vi "AlAs-GaAs superlattice-111230a.vi"() -> ()   [LabVIEW 2011]
uses:
  wait_globals.vi
panel:
  out "Total Wait Time (m:s)":string
  out "step number  2":i32
  in  "Number of \nGrowth Steps 6":i32=20
  out "Wait Time Remaining(m:s)":string
  out "Waiting":bool
  in  "Ga Flow 1":dbl=5.49
  in  "Aluminum Flow":dbl=10.0
  in  "Number of \nGrowth Steps":i32=20
  out "step number":i32
  in  "As_Gas Flow":dbl=3.4
  in  "Manifold H2 Flow":dbl=730.0
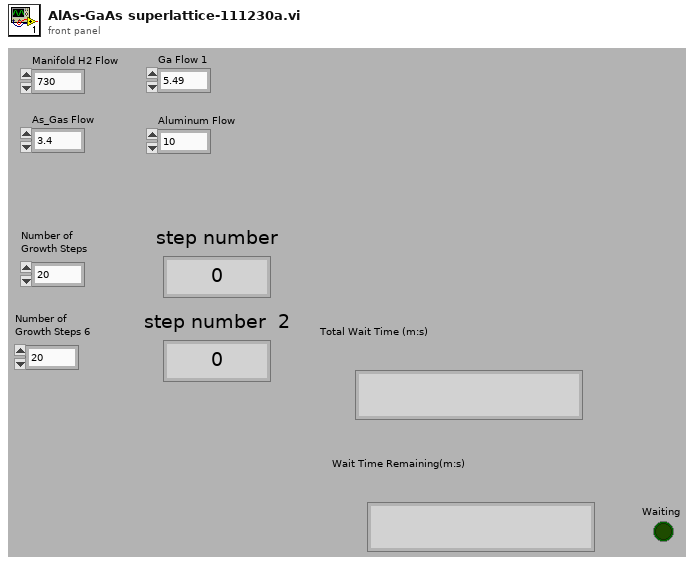
[diagram p1: front panel]
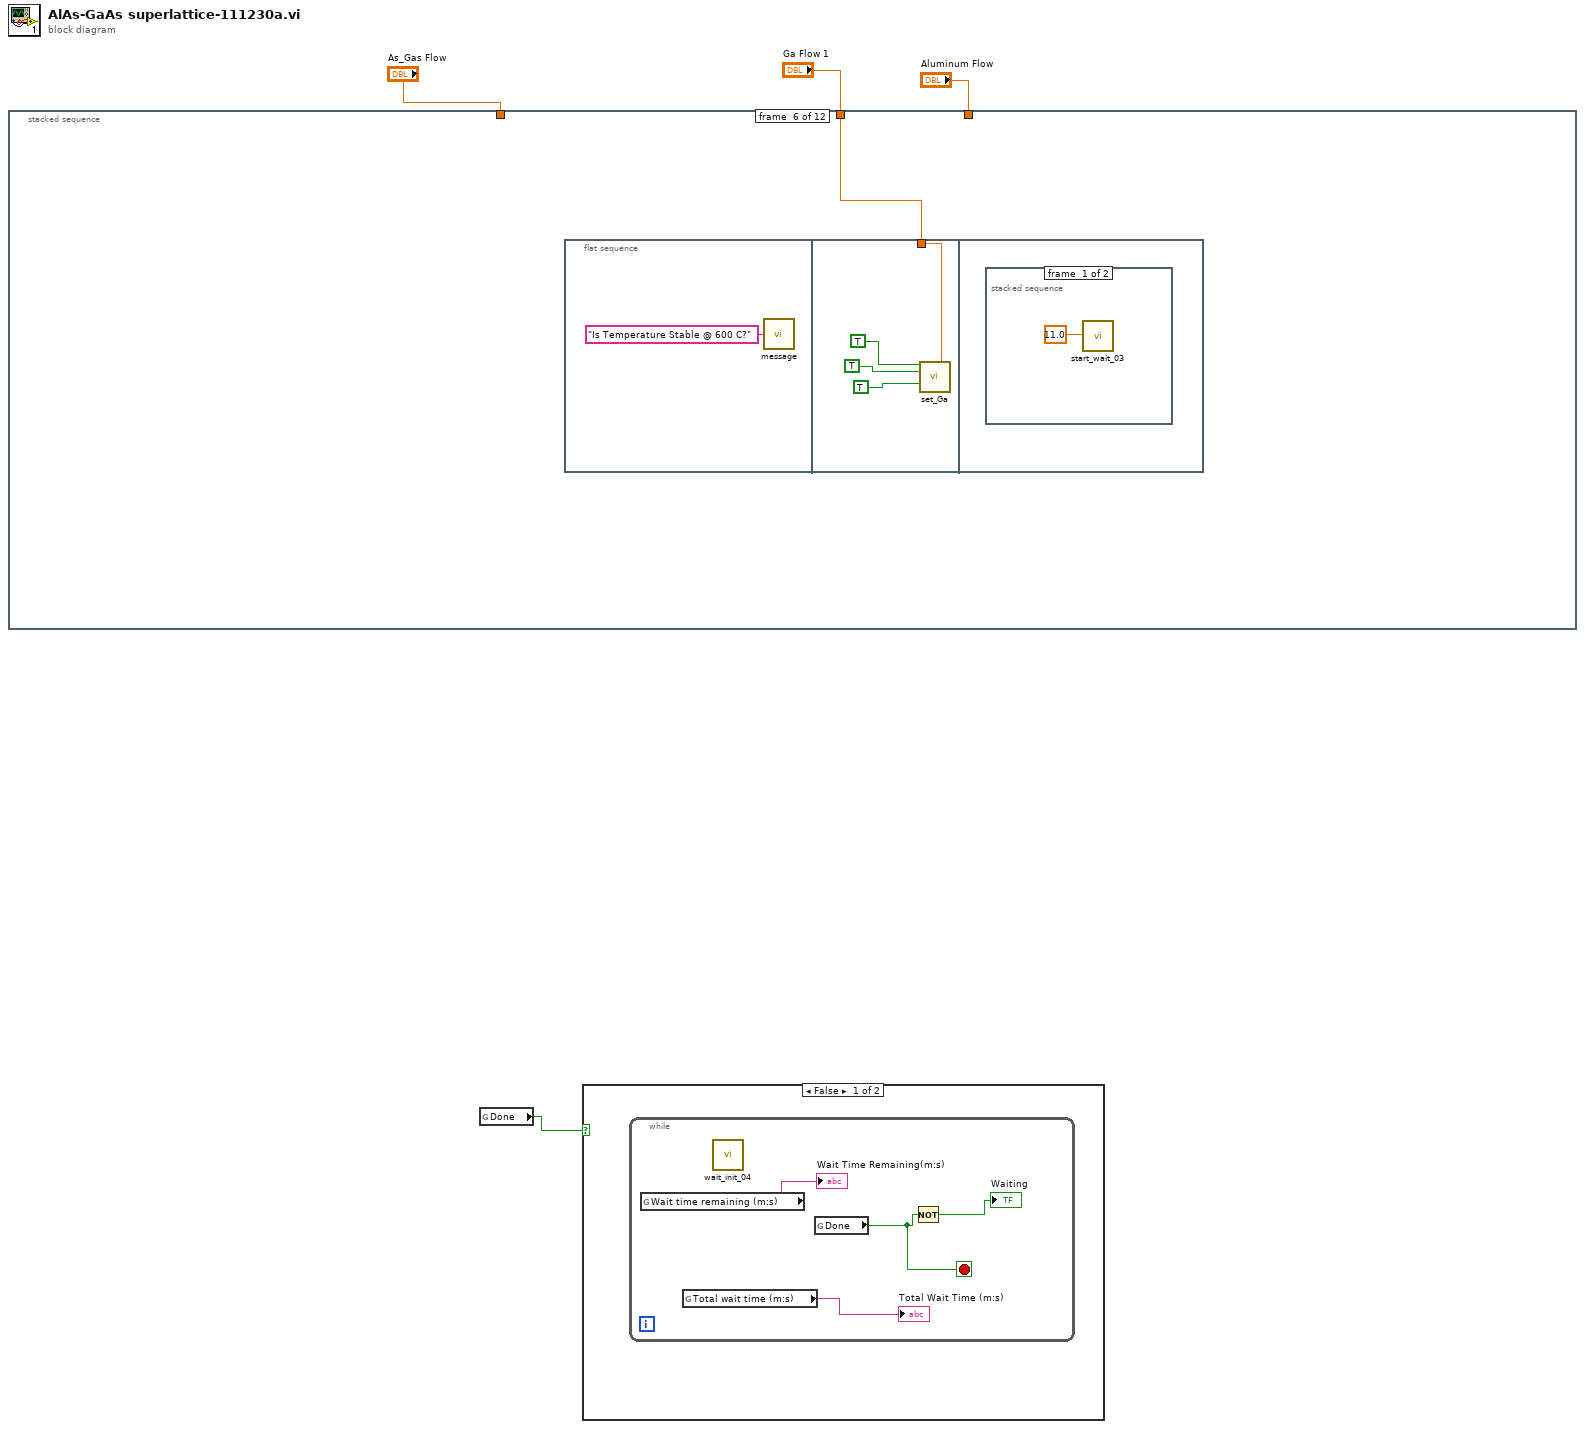
[diagram p0: block diagram]
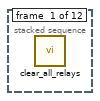
[diagram p3: hidden frame]
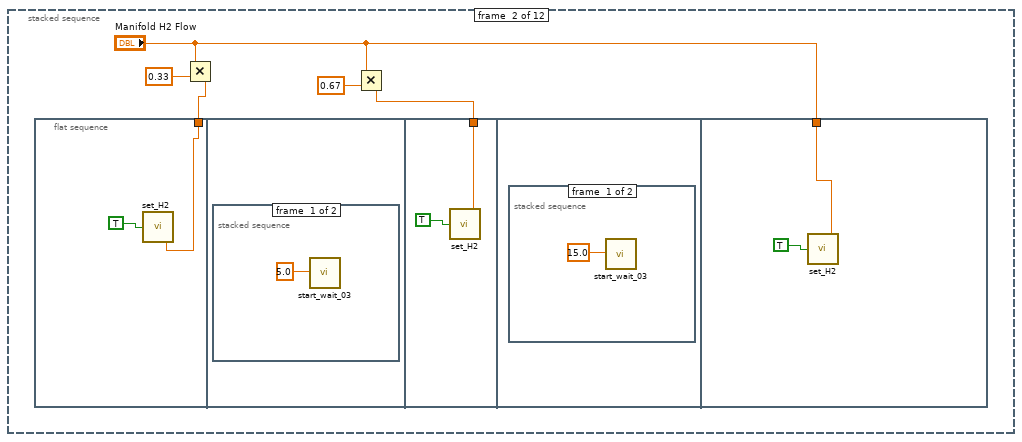
[diagram p4: hidden frame]
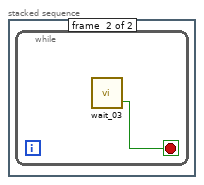
[diagram p5: hidden frame]
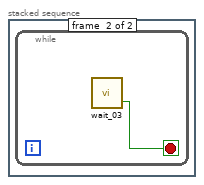
[diagram p6: hidden frame]
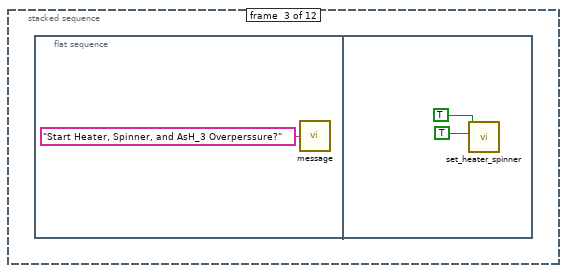
[diagram p7: hidden frame]
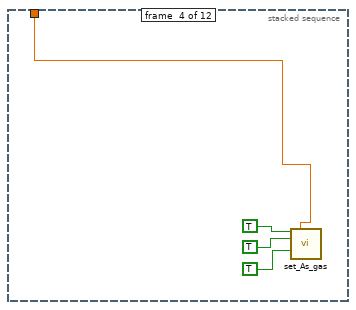
[diagram p8: hidden frame]
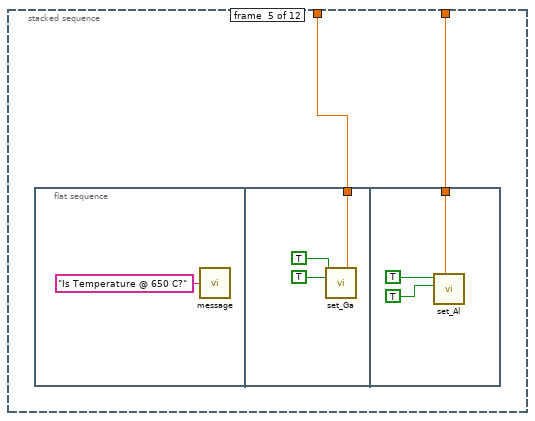
[diagram p9: hidden frame]
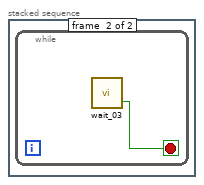
[diagram p10: hidden frame]
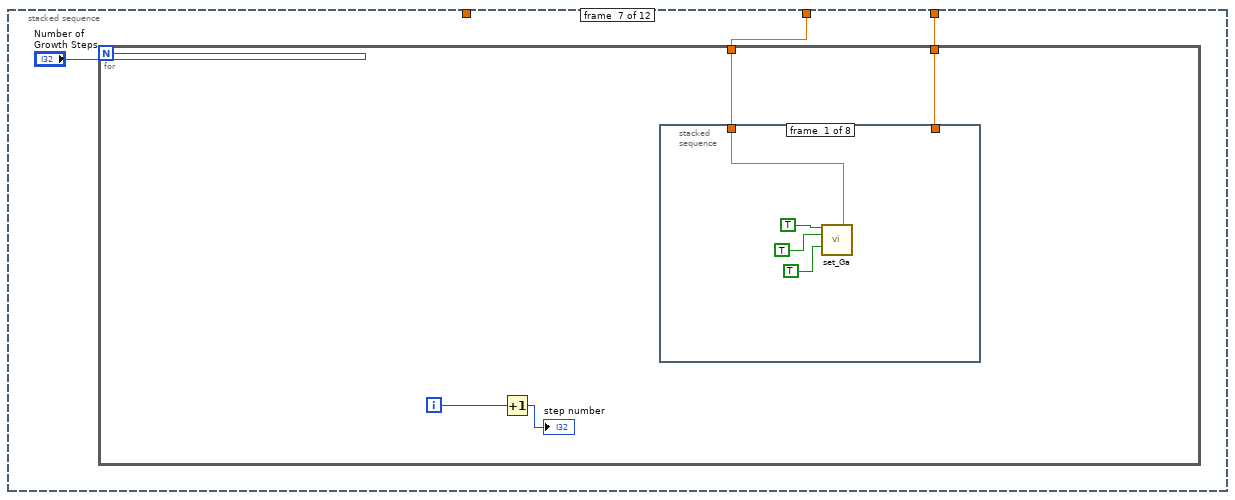
[diagram p11: hidden frame]
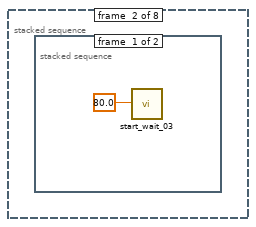
[diagram p12: hidden frame]
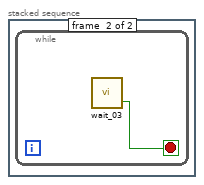
[diagram p13: hidden frame]
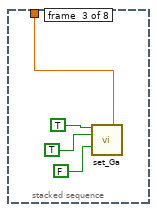
[diagram p14: hidden frame]
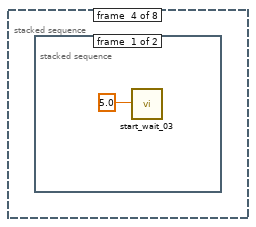
[diagram p15: hidden frame]
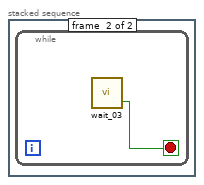
[diagram p16: hidden frame]
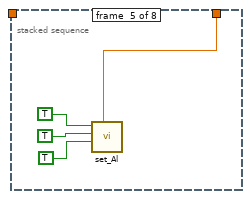
[diagram p17: hidden frame]
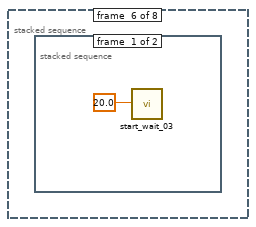
[diagram p18: hidden frame]
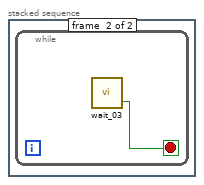
[diagram p19: hidden frame]
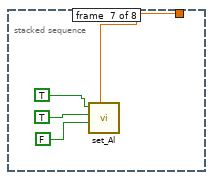
[diagram p20: hidden frame]
diagram:
  n1 = stacked-sequence {
    tunnel: "Ga Flow 1" -> [_ _ _ _ w28 w36 w45 w76 _ _ _ _]
    tunnel: "As_Gas Flow" -> [_ _ _ w23 _ _ _ _ _ _ _ _]
    tunnel: "Aluminum Flow" -> [_ _ _ _ w27 _ w44 w75 _ _ _ _]
    frame #0 {
      n2 = call "clear_all_relays.vi"() -> ()  [unwired: 2 out]
    }
    frame #1 {
      n3 = flat-sequence {
        tunnel: w9 -> [w10]
        tunnel: w7 -> [w14]
        tunnel: "Manifold H2 Flow" -> [w18]
        frame #0 {
          n4 = call "set_H2.vi"("Manifold H2 Flow"=w10, "H2 Active"=TRUE) -> ()  [unwired: 2 in, 2 out]
        }
        frame #1 {
          n5 = stacked-sequence {
            frame #0 {
              n6 = call "start_wait_03.vi"("Total wait time (s)"=5.0 ("Wait (s)")) -> ()
            }
            frame #1 {
              n7 = while {
                stop <- w13 stop-if-true
                n8 = call "wait_03.vi"() -> ("Done"=w13:bool)  [unwired: 1 in, 1 out]
              }
            }
          }
        }
        frame #2 {
          n9 = call "set_H2.vi"("Manifold H2 Flow"=w14, "H2 Active"=TRUE) -> ()  [unwired: 2 in, 2 out]
        }
        frame #3 {
          n10 = stacked-sequence {
            frame #0 {
              n11 = call "start_wait_03.vi"("Total wait time (s)"=15.0 ("Wait (s)")) -> ()
            }
            frame #1 {
              n12 = while {
                stop <- w17 stop-if-true
                n13 = call "wait_03.vi"() -> ("Done"=w17:bool)  [unwired: 1 in, 1 out]
              }
            }
          }
        }
        frame #4 {
          n14 = call "set_H2.vi"("Manifold H2 Flow"=w18, "H2 Active"=TRUE) -> ()  [unwired: 2 in, 2 out]
        }
      }
      n15 = Multiply(x="Manifold H2 Flow", y=0.33) -> (x*y=w9:dbl)
      n16 = Multiply(x="Manifold H2 Flow", y=0.67) -> (x*y=w7:dbl)
    }
    frame #2 {
      n17 = flat-sequence {
        frame #0 {
          n18 = call "message.vi"("message"="Start Heater, Spinner, and AsH_3 Overperssure?") -> ()
        }
        frame #1 {
          n19 = call "set_heater_spinner.vi"("Spinner"=TRUE, "Heater"=TRUE) -> ()  [unwired: 1 in, 7 out]
        }
      }
    }
    frame #3 {
      n20 = call "set_As_gas.vi"("As_Gas Active"=TRUE, "As_Gas Flow"=w23, "As_Gas In"=TRUE, "As_Gas Run"=TRUE) -> ()  [unwired: 2 in, 10 out]
    }
    frame #4 {
      n21 = flat-sequence {
        tunnel: w28 -> [w30]
        tunnel: w27 -> [w33]
        frame #0 {
          n22 = call "message.vi"("message"="Is Temperature @ 650 C?") -> ()
        }
        frame #1 {
          n23 = call "set_Ga.vi"("Ga Active"=TRUE, "Ga Flow 1"=w30, "Ga Bubbler"=TRUE) -> ()  [unwired: 5 in, 8 out]
        }
        frame #2 {
          n24 = call "set_Al.vi"("Aluminum Flow"=w33, "Al Bubbler"=TRUE ("Ga Bubbler"), "Al Active"=TRUE ("Ga Active")) -> ()  [unwired: 7 in]
        }
      }
    }
    frame #5 {
      n25 = flat-sequence {
        tunnel: w36 -> [w38]
        frame #0 {
          n26 = call "message.vi"("message"="Is Temperature Stable @ 600 C?") -> ()
        }
        frame #1 {
          n27 = call "set_Ga.vi"("Ga Active"=TRUE ("P_Gas Active"), "Ga Flow 1"=w38, "Ga Bubbler"=TRUE ("P_Gas In"), "Ga Run"=TRUE ("P_Gas Run")) -> ()  [unwired: 4 in, 8 out]
        }
        frame #2 {
          n28 = stacked-sequence {
            frame #0 {
              n29 = call "start_wait_03.vi"("Total wait time (s)"=11.0 ("Wait (s)")) -> ()
            }
            frame #1 {
              n30 = while {
                stop <- w43 stop-if-true
                n31 = call "wait_03.vi"() -> ("Done"=w43:bool)  [unwired: 1 in, 1 out]
              }
            }
          }
        }
      }
    }
    frame #6 {
      n32 = for {
        N: "Number of \nGrowth Steps" -> [_]
        tunnel: w45 -> [w48]
        tunnel: w44 -> [w47]
        i -> [w49]
        n33 = Increment(x=w49) -> (x+1=→"step number":i32)
        n34 = stacked-sequence {
          tunnel: w47 -> [_ _ _ _ w63 _ w70 _]
          tunnel: w48 -> [w51 _ w57 _ _ _ _ _]
          frame #0 {
            n35 = call "set_Ga.vi"("Ga Active"=TRUE ("P_Gas Active"), "Ga Flow 1"=w51, "Ga Bubbler"=TRUE ("P_Gas In"), "Ga Run"=TRUE ("P_Gas Run")) -> ()  [unwired: 4 in, 8 out]
          }
          frame #1 {
            n36 = stacked-sequence {
              frame #0 {
                n37 = call "start_wait_03.vi"("Total wait time (s)"=80.0 ("Wait (s)")) -> ()
              }
              frame #1 {
                n38 = while {
                  stop <- w56 stop-if-true
                  n39 = call "wait_03.vi"() -> ("Done"=w56:bool)  [unwired: 1 in, 1 out]
                }
              }
            }
          }
          frame #2 {
            n40 = call "set_Ga.vi"("Ga Active"=TRUE ("P_Gas Active"), "Ga Flow 1"=w57, "Ga Bubbler"=TRUE ("P_Gas In"), "Ga Run"=FALSE ("P_Gas Run")) -> ()  [unwired: 4 in, 8 out]
          }
          frame #3 {
            n41 = stacked-sequence {
              frame #0 {
                n42 = call "start_wait_03.vi"("Total wait time (s)"=5.0 ("Wait (s)")) -> ()
              }
              frame #1 {
                n43 = while {
                  stop <- w62 stop-if-true
                  n44 = call "wait_03.vi"() -> ("Done"=w62:bool)  [unwired: 1 in, 1 out]
                }
              }
            }
          }
          frame #4 {
            n45 = call "set_Al.vi"("Aluminum Flow"=w63, "Al Run"=TRUE ("P_Gas Run"), "Al Bubbler"=TRUE ("P_Gas In"), "Al Active"=TRUE ("P_Gas Active")) -> ()  [unwired: 6 in]
          }
          frame #5 {
            n46 = stacked-sequence {
              frame #0 {
                n47 = call "start_wait_03.vi"("Total wait time (s)"=20.0 ("Wait (s)")) -> ()
              }
              frame #1 {
                n48 = while {
                  stop <- w68 stop-if-true
                  n49 = call "wait_03.vi"() -> ("Done"=w68:bool)  [unwired: 1 in, 1 out]
                }
              }
            }
          }
          frame #6 {
            n50 = call "set_Al.vi"("Aluminum Flow"=w70, "Al Run"=FALSE ("P_Gas Run"), "Al Bubbler"=TRUE ("P_Gas In"), "Al Active"=TRUE ("P_Gas Active")) -> ()  [unwired: 6 in]
          }
          frame #7 {
            n51 = stacked-sequence {
              frame #0 {
                n52 = call "start_wait_03.vi"("Total wait time (s)"=5.0 ("Wait (s)")) -> ()
              }
              frame #1 {
                n53 = while {
                  stop <- w74 stop-if-true
                  n54 = call "wait_03.vi"() -> ("Done"=w74:bool)  [unwired: 1 in, 1 out]
                }
              }
            }
          }
        }
      }
    }
    frame #7 {
      n55 = for {
        N: "Number of \nGrowth Steps 6" -> [_]
        tunnel: w76 -> [w79]
        tunnel: w75 -> [w78]
        i -> [w80]
        n56 = Increment(x=w80) -> (x+1=→"step number  2":i32)
        n57 = stacked-sequence {
          tunnel: w78 -> [_ _ _ _ w94 _ w101 _]
          tunnel: w79 -> [w82 _ w88 _ _ _ _ _]
          frame #0 {
            n58 = call "set_Ga.vi"("Ga Active"=TRUE ("P_Gas Active"), "Ga Flow 1"=w82, "Ga Bubbler"=TRUE ("P_Gas In"), "Ga Run"=TRUE ("P_Gas Run")) -> ()  [unwired: 4 in, 8 out]
          }
          frame #1 {
            n59 = stacked-sequence {
              frame #0 {
                n60 = call "start_wait_03.vi"("Total wait time (s)"=80.0 ("Wait (s)")) -> ()
              }
              frame #1 {
                n61 = while {
                  stop <- w87 stop-if-true
                  n62 = call "wait_03.vi"() -> ("Done"=w87:bool)  [unwired: 1 in, 1 out]
                }
              }
            }
          }
          frame #2 {
            n63 = call "set_Ga.vi"("Ga Active"=TRUE ("P_Gas Active"), "Ga Flow 1"=w88, "Ga Bubbler"=TRUE ("P_Gas In"), "Ga Run"=FALSE ("P_Gas Run")) -> ()  [unwired: 4 in, 8 out]
          }
          frame #3 {
            n64 = stacked-sequence {
              frame #0 {
                n65 = call "start_wait_03.vi"("Total wait time (s)"=7.0 ("Wait (s)")) -> ()
              }
              frame #1 {
                n66 = while {
                  stop <- w93 stop-if-true
                  n67 = call "wait_03.vi"() -> ("Done"=w93:bool)  [unwired: 1 in, 1 out]
                }
              }
            }
          }
          frame #4 {
            n68 = call "set_Al.vi"("Aluminum Flow"=w94, "Al Run"=TRUE ("P_Gas Run"), "Al Bubbler"=TRUE ("P_Gas In"), "Al Active"=TRUE ("P_Gas Active")) -> ()  [unwired: 6 in]
          }
          frame #5 {
            n69 = stacked-sequence {
              frame #0 {
                n70 = call "start_wait_03.vi"("Total wait time (s)"=20.0 ("Wait (s)")) -> ()
              }
              frame #1 {
                n71 = while {
                  stop <- w99 stop-if-true
                  n72 = call "wait_03.vi"() -> ("Done"=w99:bool)  [unwired: 1 in, 1 out]
                }
              }
            }
          }
          frame #6 {
            n73 = call "set_Al.vi"("Aluminum Flow"=w101, "Al Run"=FALSE ("P_Gas Run"), "Al Bubbler"=TRUE ("P_Gas In"), "Al Active"=TRUE ("P_Gas Active")) -> ()  [unwired: 6 in]
          }
          frame #7 {
            n74 = stacked-sequence {
              frame #0 {
                n75 = call "start_wait_03.vi"("Total wait time (s)"=7.0 ("Wait (s)")) -> ()
              }
              frame #1 {
                n76 = while {
                  stop <- w105 stop-if-true
                  n77 = call "wait_03.vi"() -> ("Done"=w105:bool)  [unwired: 1 in, 1 out]
                }
              }
            }
          }
        }
      }
    }
    frame #8 {
      n78 = flat-sequence {
        frame #0 {
          n79 = call "set_heater_spinner.vi"("Spinner"=TRUE ("Ga Active")) -> ()  [unwired: 2 in, 7 out]
        }
        frame #1 {
          n80 = call "set_Ga.vi"("Ga Active"=TRUE, "Ga Flow 1"=10.0) -> ()  [unwired: 6 in, 8 out]
        }
        frame #2 {
          n81 = call "set_Al.vi"("Aluminum Flow"=100.0, "Al Active"=TRUE ("Ga Active")) -> ()  [unwired: 8 in]
        }
        frame #3 {
          n82 = stacked-sequence {
            frame #0 {
              n83 = call "start_wait_03.vi"("Total wait time (s)"=20.0 ("Wait (s)")) -> ()
            }
            frame #1 {
              n84 = while {
                stop <- w112 stop-if-true
                n85 = call "wait_03.vi"() -> ("Done"=w112:bool)  [unwired: 1 in, 1 out]
              }
            }
          }
        }
      }
    }
    frame #9 {
      n86 = flat-sequence {
        frame #0 {
          n87 = call "set_Ga.vi"("Ga Remote"=FALSE) -> ()  [unwired: 7 in, 8 out]
        }
        frame #1 {
          n88 = call "set_Al.vi"("Al Run"=FALSE ("Ga Remote")) -> ()  [unwired: 9 in]
        }
        frame #2 {
          n89 = call "message.vi"("message"="Is Temperature < 300C?") -> ()
        }
      }
    }
    frame #10 {
      n90 = call "set_As_gas.vi"("As_Gas Remote"=FALSE) -> ()  [unwired: 5 in, 10 out]
    }
    frame #11 {
      n91 = flat-sequence {
        frame #0 {
          n92 = call "message.vi"("message"="Is Temperarure < 100C?") -> ()
        }
        frame #1 {
          n93 = call "set_heater_spinner.vi"("Heater/Spinner Remote"=FALSE) -> ()  [unwired: 2 in, 7 out]
        }
        frame #2 {
          n94 = call "set_H2.vi"("H2N2 Remote"=FALSE) -> ()  [unwired: 3 in, 2 out]
        }
      }
    }
  }
  n95 = global read "wait_globals.vi" "Done"() -> (w1:bool)
  n96 = case shown="False" w1 {
    frame False {
    }
    frame True {
    }
  }
  n97 = while {
    stop <- w121 stop-if-true
    n98 = global read "wait_globals.vi" "Wait time remaining (m:s)"() -> (→"Wait Time Remaining(m:s)":string)
    n99 = global read "wait_globals.vi" "Total wait time (m:s)"() -> (→"Total Wait Time (m:s)":string)
    n100 = call "wait_init_04.vi"() -> ()  [unwired: 1 in]
    n101 = global read "wait_globals.vi" "Done"() -> (w121:bool)
    n102 = Not(x=w121) -> (.not. x?=→"Waiting":bool)
  }
